vi "Check if Folder exists.vi"(8 "error in (no error)":errorcluster, 11 "Exp Params in":T1={"Experiment Type"="", "Experiment Name"="", "ExpPath"=path "", "Save As"="Time Series", "TSFrames"=0, "TSfps"=0.0, "Streaming"=FALSE, "tdms ref"=refnum, "frame #"=0, "Full Path"=path "", "PeakOnQueue"=FALSE} {"TSFrames" min=1 step=1; "TSfps" min=0.001 max=90.0 step=0.001 format="%_4g"}) -> (0 "error out":errorcluster, 3 "Exp Params out":T1={"Experiment Type"="", "Experiment Name"="", "ExpPath"=path "", "Save As"="Time Series", "TSFrames"=0, "TSfps"=0.0, "Streaming"=FALSE, "tdms ref"=refnum, "frame #"=0, "Full Path"=path "", "PeakOnQueue"=FALSE} {"TSFrames" min=1 step=1; "TSfps" min=0.001 max=90.0 step=0.001 format="%_4g"})   [LabVIEW 2020]
uses:
  _controls/Exp Params.ctl
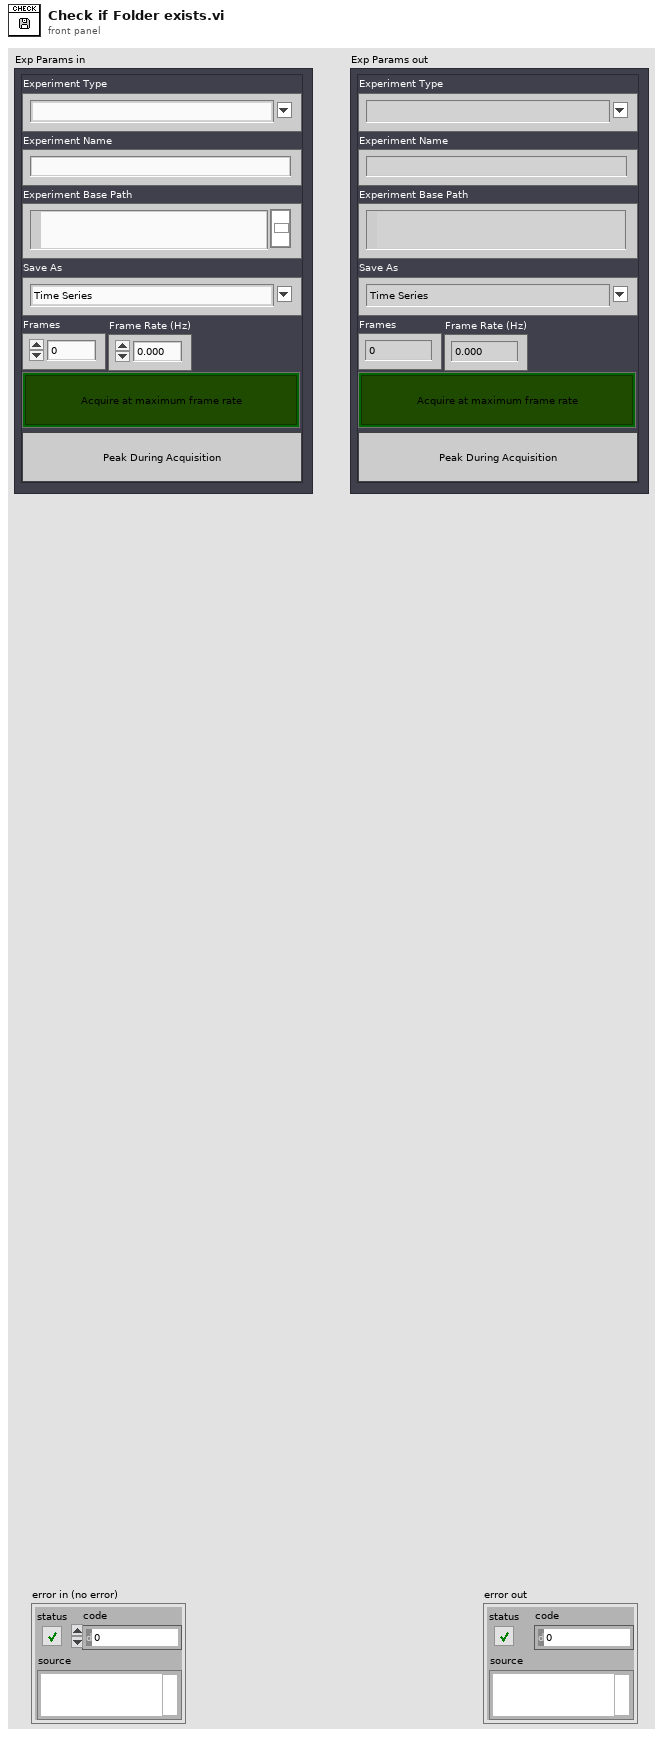
[diagram p1: front panel]
types:
  T1 = typedef "Exp Params.ctl" = cluster{"Experiment Type":string, "Experiment Name":string, "ExpPath":path, "Save As":string, "TSFrames":i32, "TSfps":dbl, "Streaming":bool, "tdms ref":refnum<k34>, "frame #":i64, "Full Path":path, "PeakOnQueue":bool}
  T2 = enum16{"open", "open or create", "create or replace", "create", "open (read-only)"}
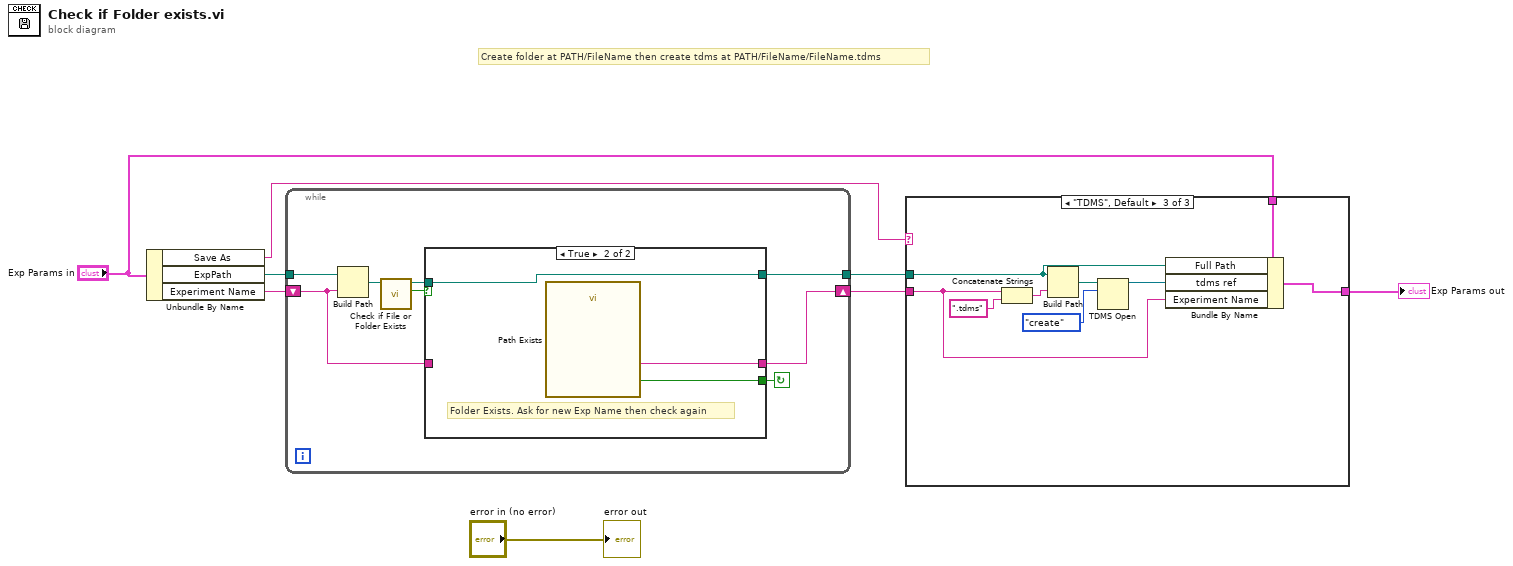
[diagram p0: block diagram]
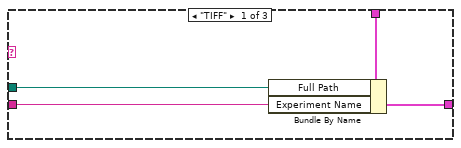
[diagram p2: hidden frame]
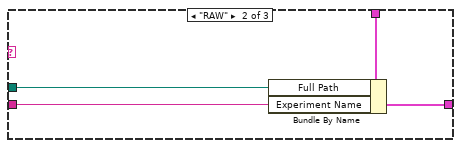
[diagram p3: hidden frame]
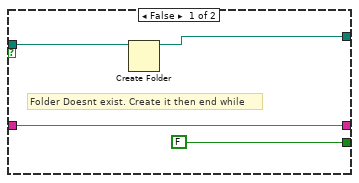
[diagram p4: hidden frame]
diagram:
  # "Create folder at PATH/FileName then create tdms at PATH/FileName/FileName.tdms"
  n1 = Unbundle By Name("Exp Params in") -> ("Save As"=w2:string, "ExpPath"=w5:path, "Experiment Name"=w7:string)
  n2 = while {
    tunnel: [w12] -> w6
    shift-right: [w10] -> w3
    shift-left: w7 -> [w9]
    tunnel: w5 -> [w11]
    stop <- w14 continue-if-true
    n3 = Build Path(base path=w11, name or relative path=w9) -> (appended path=w13:path)
    n4 = call <vilib>:"Check if File or Folder Exists.vi"("path"=w13) -> ("file or folder exists?"=w16:bool, "dup path"=w15:path)  [unwired: 8 in, 1 out]
    n5 = case shown="True" w16 {
      tunnel: w15 -> [w20 w21]
      tunnel: [FALSE ("Rename") w23] -> w14
      tunnel: [w19 w21] -> w12
      tunnel: [w18 w22] -> w10
      tunnel: w9 -> [w18 _]
      frame False {
        # "Folder Doesnt exist. Create it then end while"
        n6 = Create Folder(path (use dialog)=w20) -> (created path=w19:path)  [unwired: 2 in, 2 out]
      }
      frame True {
        # "Folder Exists. Ask for new Exp Name then check again"
        n7 = call "Path Exists"() -> ("NewName"=w22:string, "Rename"=w23:bool)  [unwired: 17 in, 1 out]
      }
    }
  }
  n8 = case shown="\"TDMS\", Default" w2 {
    tunnel: w6 -> [w24 w28 w32]
    tunnel: [w26 w30 w35] -> w1
    tunnel: "Exp Params in" -> [w27 w31 w34]
    tunnel: w3 -> [w25 w29 w33]
    frame "TIFF" {
      n9 = Bundle By Name(cluster=w27, "Full Path"=w24, "Experiment Name"=w25) -> (w26:T1)
    }
    frame "RAW" {
      n10 = Bundle By Name(cluster=w31, "Full Path"=w28, "Experiment Name"=w29) -> (w30:T1)
    }
    frame "TDMS", Default {
      n11 = Concatenate Strings(w33, ".tdms" ("string")) -> (w38:string)
      n12 = Build Path(base path=w32, name or relative path=w38) -> (appended path=w37:path)
      n13 = TDMS Open(10:T2."create" ("operation (0:open)"), 11:w37) -> (3:w39:refnum<k34>)  [unwired: 5 in, 1 out]
      n14 = Bundle By Name(cluster=w34, "Full Path"=w32, "tdms ref"=w39, "Experiment Name"=w33) -> (w35:T1)
    }
  }
  "Exp Params out" <- w1
  "error out" <- "error in (no error)"
